vi "ROS_Master_CantDoThat.vi"() -> (0 "XML":string)   [LabVIEW 2012]
doc: "Returns an error for unsupported topics"
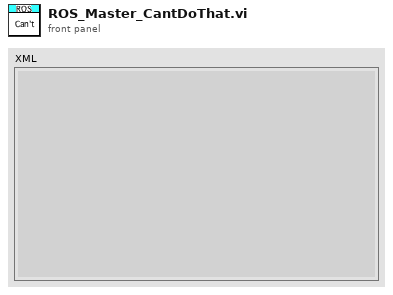
[diagram p1: front panel]
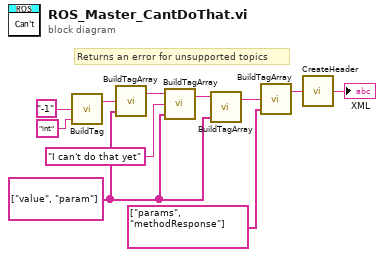
[diagram p0: block diagram]
diagram:
  w1 = string[] ["value", "param"] ("tags")
  # "Returns an error for unsupported topics"
  n1 = call <userlib>:"BuildTag.vi"("tag"="int", "value"="-1") -> ("string out"=w7:string)  [unwired: 2 in]
  n2 = call <userlib>:"BuildTagArray.vi"("tags"=w1, "value"=w7) -> ("string out"=w2:string)  [unwired: 2 in]
  n3 = call <userlib>:"BuildTagArray.vi"("tags"=w1, "value"="I can't do that yet", "string in"=w2) -> ("string out"=w3:string)  [unwired: 1 in]
  n4 = call <userlib>:"BuildTagArray.vi"("tags"=w1, "string in"=w3) -> ("string out"=w9:string)  [unwired: 2 in]
  n5 = call <userlib>:"BuildTagArray.vi"("tags"=string[] ["params", "methodResponse"], "value"=w9) -> ("string out"=w10:string)  [unwired: 2 in]
  n6 = call <userlib>:"CreateHeader.vi"("Content"=w10) -> ("XML"=→"XML":string)
